vi "Ballard - 1553 - Load Parameters File.vi"(8 "error in (no error)":errorcluster, 11 "Node Ptr":u64 format="%.0x") -> (0 "error out":errorcluster)   [LabVIEW 2020, in "Ballard 1553 System Explorer.lvlib"]
uses:
  Ballard 1553 System Explorer.lvlib
  Shared/Controls and Global/Global.vi
  <vilib>/NI VeriStand/Custom Device API/Get Item Property (Path).vi
  <vilib>/NI VeriStand/Custom Device API/Set Item Property (String).vi
  <vilib>/NI VeriStand/Custom Device API/Set Item Property (Path).vi
  <vilib>/NI VeriStand/Custom Device API/Custom Device API.lvlib
  <vilib>/NI VeriStand/Custom Device Tools/Custom Device Utility Library/Custom Device Utility Library.lvlib
  Shared/Ballard 1553 Shared.lvlib
panel:
  in  "Tag":string
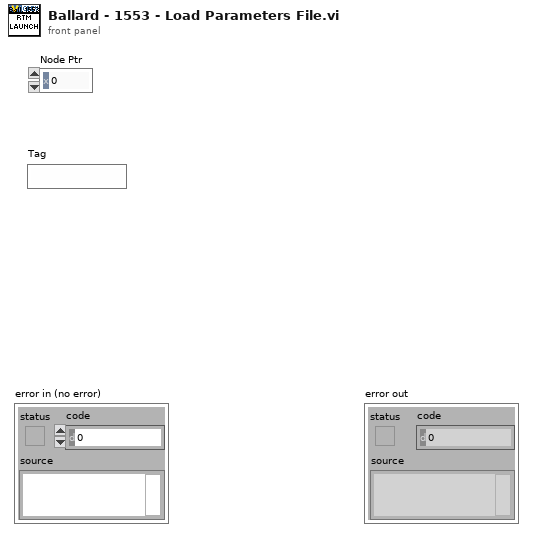
[diagram p1: front panel]
types:
  T1 = typedef "Custom Device API.lvlib/Custom Device Item Ref.ctl" = u64
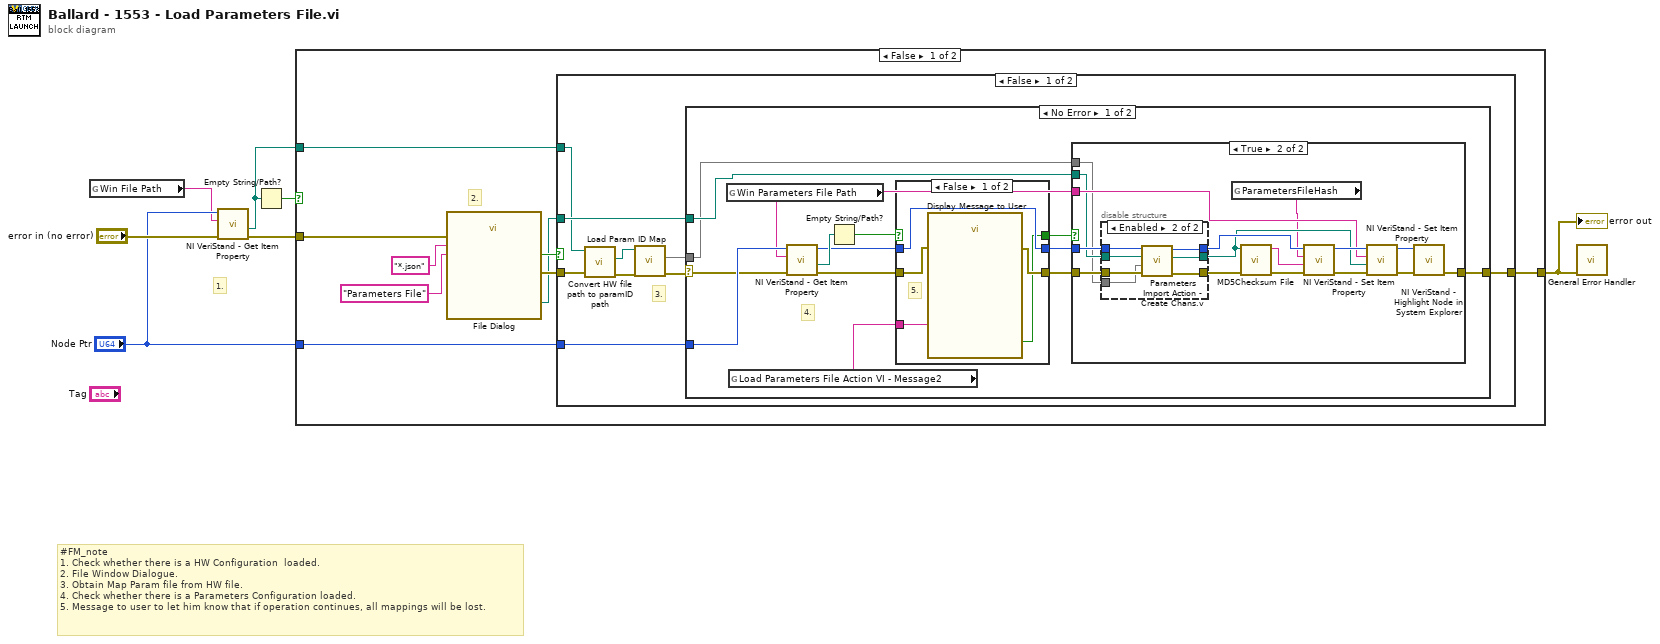
[diagram p0: block diagram]
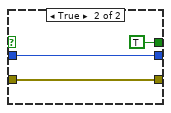
[diagram p2: hidden frame]
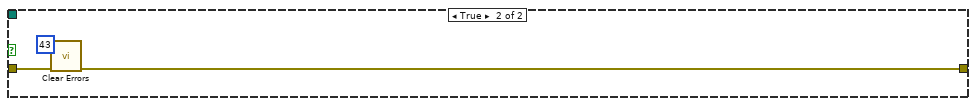
[diagram p6: hidden frame]
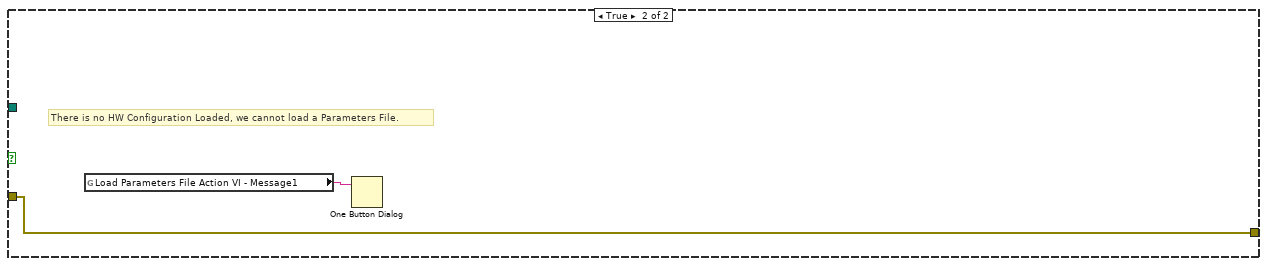
[diagram p7: hidden frame]
diagram:
  # "#FM_note \n1. Check whether there is a HW Configuration  loaded.\n2. File Window Dialogue.\n3. Obtain Map Param file from HW file.\n4. Check whether there is a Parameters Configuration loaded.\n5. Message to user to let him know that if operation continues, all mappings will be lost."
  # "1."
  n1 = global read "Global.vi" "Win File Path"() -> (w2:string)
  n2 = call-poly <vilib>:"NI VeriStand - Get Item Property.vi"("error in (no error)"="error in (no error)", "Property Name"=w2, "Item Ref in"="Node Ptr") -> ("error out"=w4:errorcluster, "Value"=w1:path)  [unwired: 5 in, 2 out]
  n3 = Empty String/Path?(string/path=w1) -> (empty?=w3:bool)
  n4 = case shown="False" w3 {
    tunnel: [w16 w80] -> w7
    tunnel: "Node Ptr" -> [w10 _]
    tunnel: w4 -> [w9 w80]
    tunnel: w1 -> [w8 _]
    frame False {
      # "2."
      n5 = call "File Dialog"("error in"=w9, "pattern (all files)"="*.json", "pattern label"="Parameters File") -> ("selected path"=w11:path, "cancelled"=w13:bool, "error out"=w12:errorcluster)  [unwired: 9 in, 1 out]
      n6 = case shown="False" w13 {
        tunnel: [w25 w77] -> w16
        tunnel: w12 -> [w22 w78]
        tunnel: w10 -> [w24 _]
        tunnel: w11 -> [w23 _]
        tunnel: w8 -> [w21 _]
        frame False {
          # "3."
          n7 = call "Convert HW file path to paramID path.vi"("error in (no error)"=w22, "Hw File In"=w21) -> ("error out"=w19:errorcluster, "Param Id File out"=w20:path)  [unwired: 7 in, 1 out]
          n8 = call "Load Param ID Map.vi"("error in (no error)"=w19, "Param Id File in"=w20) -> ("error out"=w18:errorcluster, "Param ID map"=w17:map{i32, string})  [unwired: 7 in, 1 out]
          n9 = case shown="No Error" w18 {
            selector: w18 -> [w36 w75]
            tunnel: [w39 w75] -> w25
            tunnel: w24 -> [w38 _]
            tunnel: w23 -> [w29 _]
            tunnel: w17 -> [w26 _]
            frame No Error {
              # "4."
              n10 = global read "Global.vi" "Win Parameters File Path"() -> (w28:string)
              n11 = global read "Global.vi" "Load Parameters File Action VI - Message2"() -> (w27:string)
              n12 = call-poly <vilib>:"NI VeriStand - Get Item Property.vi"("error in (no error)"=w36, "Property Name"=w28, "Item Ref in"=w38) -> ("error out"=w34:errorcluster, "Value"=w37:path, "Item Ref out"=w33:T1)  [unwired: 5 in, 1 out]
              n13 = Empty String/Path?(string/path=w37) -> (empty?=w35:bool)
              n14 = case shown="False" w35 {
                tunnel: w34 -> [w43 w46]
                tunnel: w33 -> [w44 w45]
                tunnel: [w41 TRUE] -> w32
                tunnel: [w42 w46] -> w31
                tunnel: [w44 w45] -> w30
                tunnel: w27 -> [w40 _]
                frame False {
                  # "5."
                  n15 = call "Display Message to User"("error in (no error)"=w43, "Message"=w40) -> ("error out"=w42:errorcluster, "OK"=w41:bool)  [unwired: 8 in]
                }
                frame True {
                }
              }
              n16 = case shown="True" w32 {
                tunnel: [w48 w64] -> w39
                tunnel: w28 -> [_ w57]
                tunnel: w31 -> [w48 w55]
                tunnel: w30 -> [_ w56]
                tunnel: w29 -> [_ w52]
                tunnel: w26 -> [_ w49]
                frame False {
                }
                frame True {
                  n17 = disable-structure shown="Enabled" {
                    disable-tunnel: w56 -> [w65 w72]
                    disable-tunnel: w55 -> [w67 w74]
                    disable-tunnel: [w65 w69] -> w54
                    disable-tunnel: [w67 w71] -> w53
                    disable-tunnel: w52 -> [w66 w73]
                    disable-tunnel: [w66 w70] -> w51
                    disable-tunnel: w49 -> [_ w68]
                    frame Disabled {
                    }
                    frame Enabled {
                      n18 = call "Parameters Import Action - Create Chans.v.vi"("error in (no error)"=w74, "Param ID map"=w68, "selected path"=w73, "Item Ref in"=w72) -> ("error out"=w71:errorcluster, "selected path out"=w70:path, "Item Ref out"=w69:T1)  [unwired: 5 in]
                    }
                  }
                  n19 = global read "Global.vi" "ParametersFileHash"() -> (w50:string)
                  n20 = call <vilib>:"MD5Checksum File.vi"("error in (no error)"=w53, "Path"=w51) -> ("error out"=w59:errorcluster, "MD5 message-digest"=w58:string)  [unwired: 8 in]
                  n21 = call-poly <vilib>:"NI VeriStand - Set Item Property.vi"("error in (no error)"=w59, "Value"=w58, "Property Name"=w50, "Item Ref in"=w54) -> ("error out"=w60:errorcluster, "Item Ref out"=w61:T1)  [unwired: 5 in, 1 out]
                  n22 = call-poly <vilib>:"NI VeriStand - Set Item Property.vi"("error in (no error)"=w60, "Value"=w51, "Property Name"=w57, "Item Ref in"=w61) -> ("error out"=w63:errorcluster, "Item Ref out"=w62:T1)  [unwired: 5 in, 1 out]
                  n23 = call <vilib>:"NI VeriStand - Highlight Node in System Explorer.vi"("error in (no error)"=w63, "Item Ref in"=w62) -> ("error out"=w64:errorcluster)  [unwired: 8 in, 1 out]
                }
              }
            }
            frame Error {
            }
          }
        }
        frame True {
          n24 = call <vilib>:"Clear Errors.vi"("error in (no error)"=w78, "specific error code to clear (0: all)"=43) -> ("error out"=w77:errorcluster)  [unwired: 4 in, 1 out]
        }
      }
    }
    frame True {
      # "There is no HW Configuration Loaded, we cannot load a Parameters File."
      n25 = global read "Global.vi" "Load Parameters File Action VI - Message1"() -> (w79:string)
      n26 = One Button Dialog(message=w79) -> ()  [unwired: 1 in, 1 out]
    }
  }
  "error out" <- w7
  n27 = call <vilib>:"General Error Handler.vi"("error in (no error)"=w7) -> ()  [unwired: 10 in, 5 out]
